vi "Host - Get HW Config.vi"(8 "error in (no error)":errorcluster, 11 "serverName":string="10.0.18.244") -> (0 "error out":errorcluster, 3 "HW Config":T1)   [LabVIEW 2016, in "Scan Engine Custom Device.lvlib"]
uses:
  Scan Engine Custom Device.lvlib
  Type Defs/Host - Module.ctl
  Type Defs/Host - Slave.ctl
  Type Defs/Host - Master.ctl
  Type Defs/Host - HW Config.ctl
  Type Defs/Host - Local Chassis.ctl
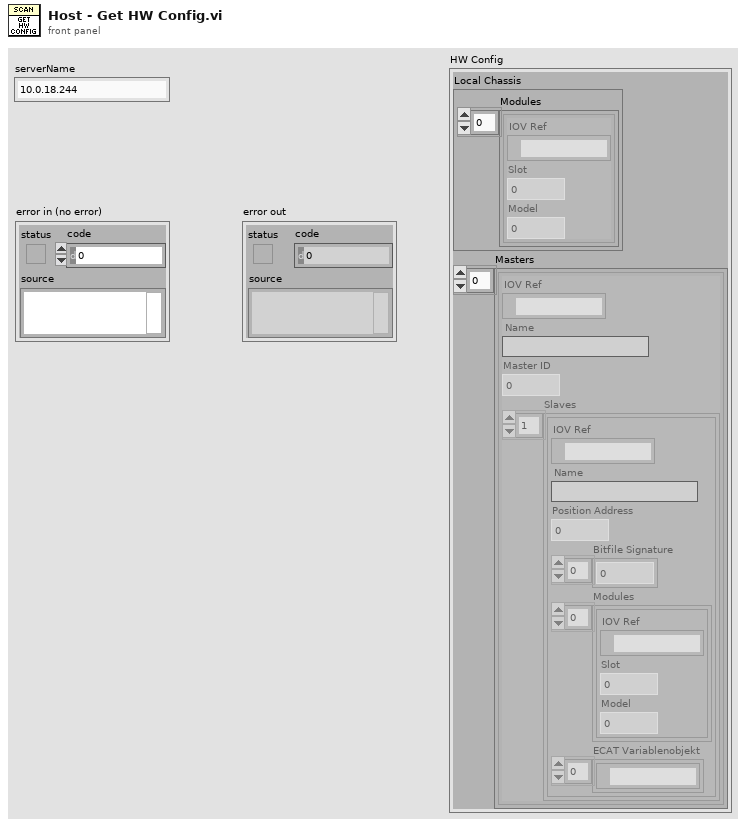
[diagram p1: front panel]
types:
  T1 = typedef "Scan Engine Custom Device.lvlib/Host - HW Config.ctl" = cluster{"Local Chassis":T2, "Masters":T4[]}
  T2 = typedef "Scan Engine Custom Device.lvlib/Host - Local Chassis.ctl" = cluster{"Modules":T3[]}
  T3 = typedef "Scan Engine Custom Device.lvlib/Host - Module.ctl" = cluster{"IOV Ref":refnum<k21>, "Slot":u32, "Model":u32}
  T4 = typedef "Scan Engine Custom Device.lvlib/Host - Master.ctl" = cluster{"IOV Ref":refnum<k21>, "Name":string, "Master ID":u32, "Slaves":T5[]}
  T5 = typedef "Scan Engine Custom Device.lvlib/Host - Slave.ctl" = cluster{"IOV Ref":refnum<k21>, "Name":string, "Position Address":u16, "Bitfile Signature":u8[], "Modules":T3[], "ECAT Variablenobjekt":refnum<k21>[]}
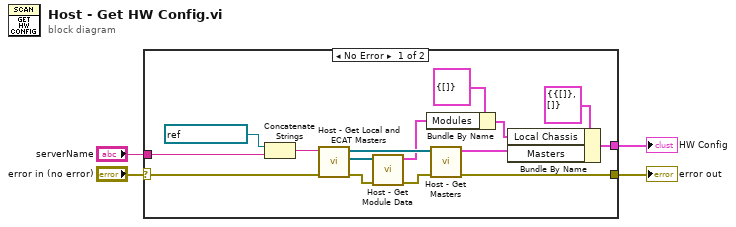
[diagram p0: block diagram]
diagram:
  n1 = case shown="No Error" "error in (no error)" {
    selector: "error in (no error)" -> [w16 w20]
    tunnel: "serverName" -> [w18 _]
    tunnel: [w14 w20] -> w3
    tunnel: [w10 _] -> w1
    frame No Error {
      n2 = Concatenate Strings(refnum<k21> "ni.var.io://" ("IOV Engine in"), w18) -> (w15:string)
      n3 = call "Host - Get Local and ECAT Masters.vi"("error in (no error)"=w16, "Refnum in"=w15) -> ("error out"=w9:errorcluster, "All Local Mods"=w13:refnum<k21>[], "All ECAT Masters"=w17:refnum<k21>[])  [unwired: 6 in, 1 out]
      n4 = call "Host - Get Module Data.vi"("error in (no error)"=w9, "Mod IOVs"=w13) -> ("error out"=w8:errorcluster, "Modules"=w6:T3[])  [unwired: 8 in]
      n5 = Bundle By Name(cluster=T2 {"Modules"=[]} ("Local Chassis"), "Modules"=w6) -> (w5:T2)
      n6 = call "Host - Get Masters.vi"("error in (no error)"=w8, "All ECAT Masters"=w17) -> ("error out"=w14:errorcluster, "Array"=w11:T4[])  [unwired: 8 in]
      n7 = Bundle By Name(cluster=T1 {"Local Chassis"={"Modules"=[]}, "Masters"=[]} ("HW Config"), "Local Chassis"=w5, "Masters"=w11) -> (w10:T1)
    }
    frame Error {
    }
  }
  "error out" <- w3
  "HW Config" <- w1
